vi "sub_update_next_state.vi"(11 "current_state":bool[][](array[boolean])) -> (3 "next state":bool[][](array[boolean]))   [LabVIEW 2018]
uses:
  index.ctl
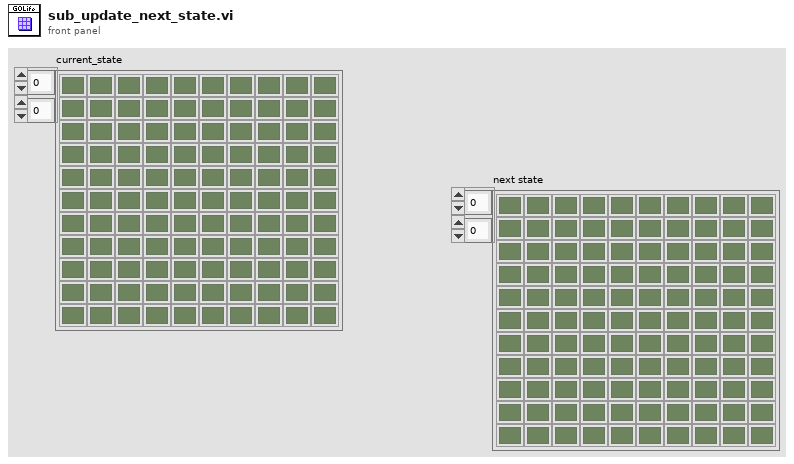
[diagram p1: front panel]
types:
  T1 = typedef "index.ctl" = cluster{"row":i32, "col":i32, "state":bool}
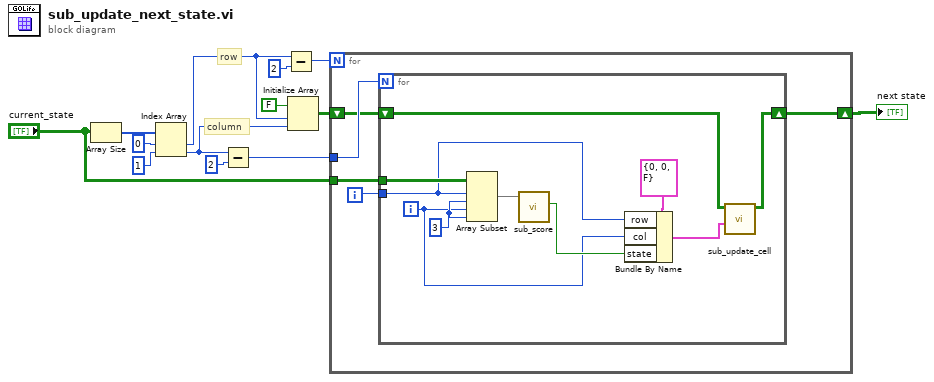
[diagram p0: block diagram]
diagram:
  # "column"
  # "row"
  n1 = Array Size(array="current_state") -> (size(s)=w13:i32[])
  n2 = Index Array(array=w13, index #1=0 ("index"), index #2=1 ("index")) -> (element #1=w6:i32, element #2=w4:i32)
  n3 = Subtract(x=w4, y=2) -> (x-y=w2:i32)
  n4 = Subtract(x=w6, y=2) -> (x-y=w7:i32)
  n5 = Initialize Array(FALSE, w6, w4) -> (w9:bool[][])
  n6 = for {
    N: w7 -> [_]
    tunnel: w2 -> [w18]
    shift-right: [w14] -> w1
    shift-left: w9 -> [w15]
    tunnel: "current_state" -> [w17]
    i -> [w16]
    n7 = for {
      N: w18 -> [_]
      tunnel: w17 -> [w28]
      tunnel: w16 -> [w23]
      shift-right: [w20] -> w14
      shift-left: w15 -> [w21]
      i -> [w22]
      w27 = 3
      n8 = Array Subset(array=w28, index (row)=w23, length (row)=w27, index (col)=w22, length (col)=w27) -> (w26:bool[][])
      n9 = call "sub_score.vi"("Array In"=w26) -> ("next state"=w24:bool)  [unwired: 9 in, 1 out]
      n10 = Bundle By Name(cluster=T1 {"row"=0, "col"=0, "state"=FALSE} ("state"), "row"=w23, "col"=w22, "state"=w24) -> (w19:T1)
      n11 = call "sub_update_cell.vi"("state"=w19, "Array In"=w21) -> ("Array Out"=w20:bool[][])  [unwired: 8 in, 1 out]
    }
  }
  "next state" <- w1
